vi "Calibrate Wavelength.vi"() -> ()   [LabVIEW 2016]
panel:
  in  "Spectrum file":path
  in  "Done":bool
  in  "nm/pixel":dbl=0.054 step=0.001
  in  "Start wavelength":dbl=400.0
  out "XY Graph":cluster{"Array - Numeric":dbl[], dbl[]}[](graph)
  out "max value":dbl format="%#_6p"
  out "error out":errorcluster
  in  "error in (no error)":errorcluster
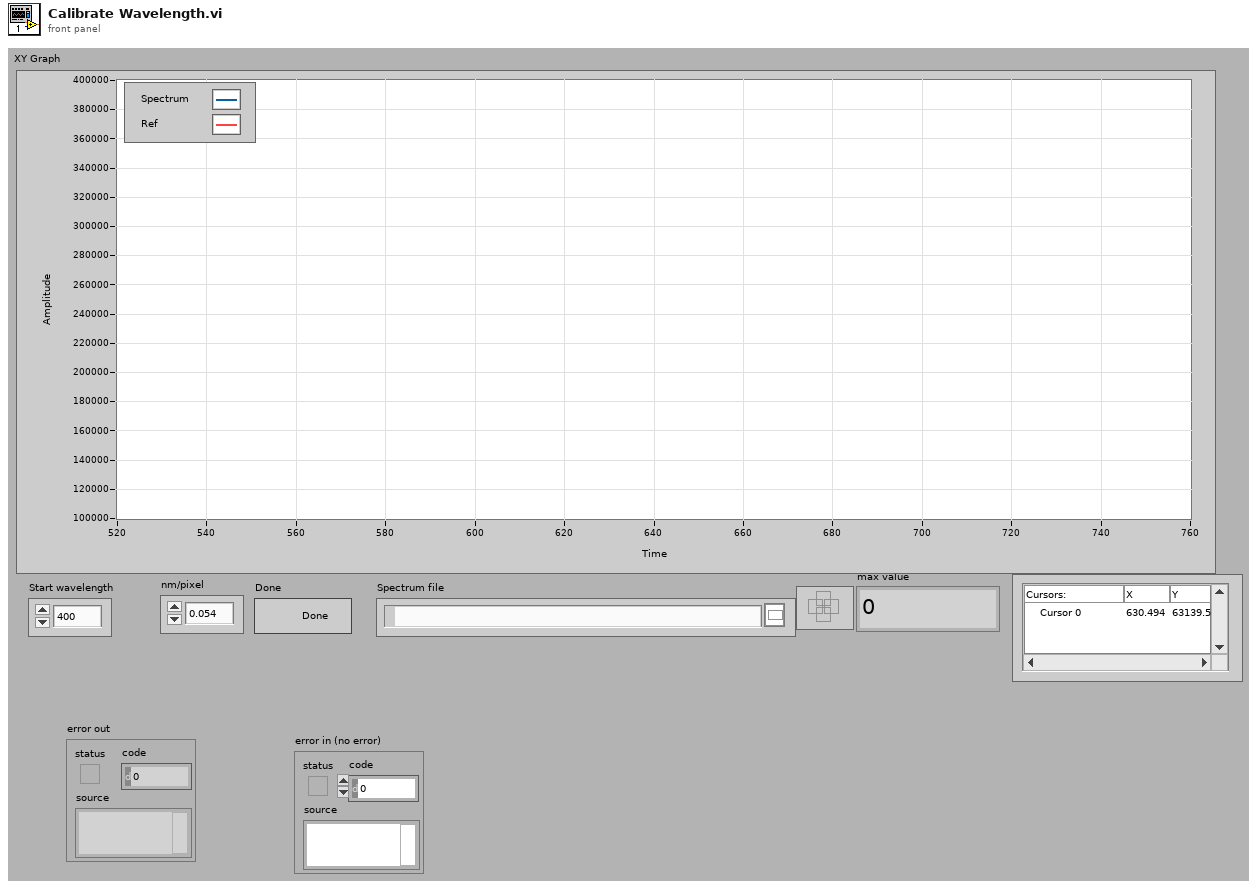
[diagram p1: front panel]
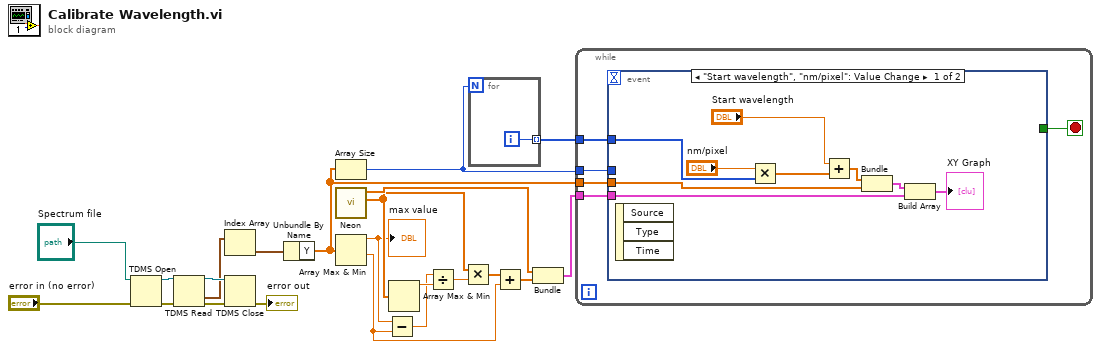
[diagram p0: block diagram]
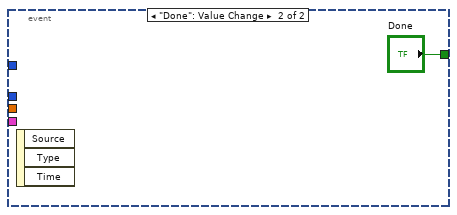
[diagram p2: hidden frame]
diagram:
  n1 = TDMS Open(8:"error in (no error)", 11:"Spectrum file") -> (0:w9:errorcluster, 3:w7:refnum<k34>)  [unwired: 5 in]
  n2 = TDMS Read(0:w7, 11:w9) -> (4:w6:refnum<k34>, 10:w5:waveform(dbl)[], 15:w10:errorcluster)  [unwired: 6 in, 3 out]
  n3 = Index Array(array=w5) -> (element=w4:waveform(dbl))  [unwired: 1 in]
  n4 = TDMS Close(8:w10, 11:w6) -> (0:→"error out":errorcluster)  [unwired: 1 out]
  n5 = Unbundle By Name(w4) -> ("Y"=w2:dbl[])
  n6 = Array Size(array=w2) -> (size(s)=w22:i32)
  n7 = call "Neon.vi"() -> ("Array - Numeric 2"=w17:dbl[], "Array - Numeric"=w20:dbl[])  [unwired: 10 in]
  n8 = Array Max & Min(array=w2) -> (max value=w14:dbl, min value=w11:dbl)  [unwired: 2 out]
  "max value" <- w14
  n9 = Subtract(x=w14, y=w11) -> (x-y=w13:dbl)
  n10 = Array Max & Min(array=w17) -> (max value=w19:dbl)  [unwired: 3 out]
  n11 = Divide(x=w13, y=w19) -> (x/y=w18:dbl)
  n12 = Multiply(x=w17, y=w18) -> (x*y=w16:dbl[])
  n13 = for {
    N: w22 -> [_]
    tunnel: [w23] -> w21 mode=indexing
    i -> [w23]
  }
  n14 = Add(x=w16, y=w11) -> (x+y=w12:dbl[])
  n15 = Bundle("Array - Numeric"=w20, w12) -> (w15:cluster{"Array - Numeric":dbl[], dbl[]})  [unwired: 1 in]
  n16 = while {
    tunnel: w22 -> [w28]
    tunnel: w21 -> [w27]
    tunnel: w2 -> [w26]
    tunnel: w15 -> [w25]
    stop <- w24 stop-if-true
    n17 = event shown="[0] \"Start wavelength\", \"nm/pixel\": Value Change" {
      selector: _ -> [_ _]
      dyn-events: _ -> [_ _]
      timeout: _ -> [_ _]
      tunnel: w28 -> [_ _]
      tunnel: w27 -> [w37 _]
      tunnel: w26 -> [w34 _]
      tunnel: w25 -> [w32 _]
      tunnel: [_ "Done"] -> w24
      event "Start wavelength", "nm/pixel": Value Change {
        n18 = event-data() -> ()  [unwired: 1 in, 3 out]
        n19 = Multiply(x="nm/pixel", y=w37) -> (x*y=w36:dbl[])
        n20 = Add(x="Start wavelength", y=w36) -> (x+y=w35:dbl[])
        n21 = Bundle(w35, "Y"=w34) -> (w33:cluster{dbl[], "Y":dbl[]})  [unwired: 1 in]
        n22 = Build Array(w33, w32) -> (→"XY Graph":cluster{"Array - Numeric":dbl[], "Y":dbl[]}[])
      }
      event "Done": Value Change {
        n23 = event-data() -> ()  [unwired: 1 in, 3 out]
      }
    }
  }
